vi "PH_TKTDS-30xx.contents.vi"   [LabVIEW 2014, in "PH_TKTDS-30xx.lvlib"]
doc: "This class is forseen to xxx\n\nThis class is part of the PHELIX xxx layer."
uses:
  PH_TKTDS-30xx.lvlib
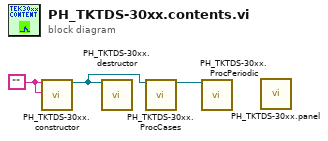
[diagram p0: block diagram]
diagram:
  w1 = ""
  n1 = call "PH_TKTDS-30xx.constructor.vi"("name"=w1, "data in"=w1) -> ("i ref out"=w2:refnum<vi>)  [unwired: 15 in, 2 out]
  n2 = call "PH_TKTDS-30xx.destructor.vi"("i ref in"=w2) -> ()  [unwired: 18 in, 1 out]
  n3 = call "PH_TKTDS-30xx.ProcCases.vi"("i ref in"=w2) -> ("i ref out"=w3:refnum<vi>)  [unwired: 16 in, 2 out]
  n4 = call "PH_TKTDS-30xx.ProcPeriodic.vi"("i ref in"=w3) -> ()  [unwired: 16 in, 3 out]
  n5 = call "PH_TKTDS-30xx.panel.vi"() -> ()  [unwired: 19 in, 1 out]
